vi "RQST Wait on Multiple Requests.vi"(6 "Processed Outgoing":refnum<queue>, 7 "Name":string, 8 "error in (no error)":errorcluster, 9 "value":T4[](array[typedef]), 10 "Source Address":u8=27, 11 "RQST ref":T3) -> (0 "error out":errorcluster, 1 "Global Requests":bool[](array[boolean]), 2 "Timeouts":bool[](array[boolean]), 3 "Elements":T1[](array[typedef]) {"payload" format="%x"; "timestamp" format="%<%.7X\n%x>T"; "type" items=["CAN Data"=0, "CAN Remote"=1, "CAN Bus Error"=2, "J1939 Data"=192, "Delay"=224, "Log Trigger"=225, "Start Trigger"=226]; "identifier" format="%x"})   [LabVIEW 2013, in "J1939.lvlib"]
uses:
  J1939.lvlib
  API Types/WS_Request Message.ctl
  RQST Lookup Table Reference.ctl
  <vilib>/xnet/xnet.llb/XNET Frame CAN.ctl
  <vilib>/xnet/xnet.llb/XNET Frame Type CAN.ctl
  API Types/CAN Outgoing Message Cluster.ctl
  RQST Lookup Table Cluster.ctl
  Common Messages/J1939 Message Request.vi
  Frame Conversion/Common Conversions.vi
  Frame Conversion/Convert J1939 ID to CAN Arb ID.vi
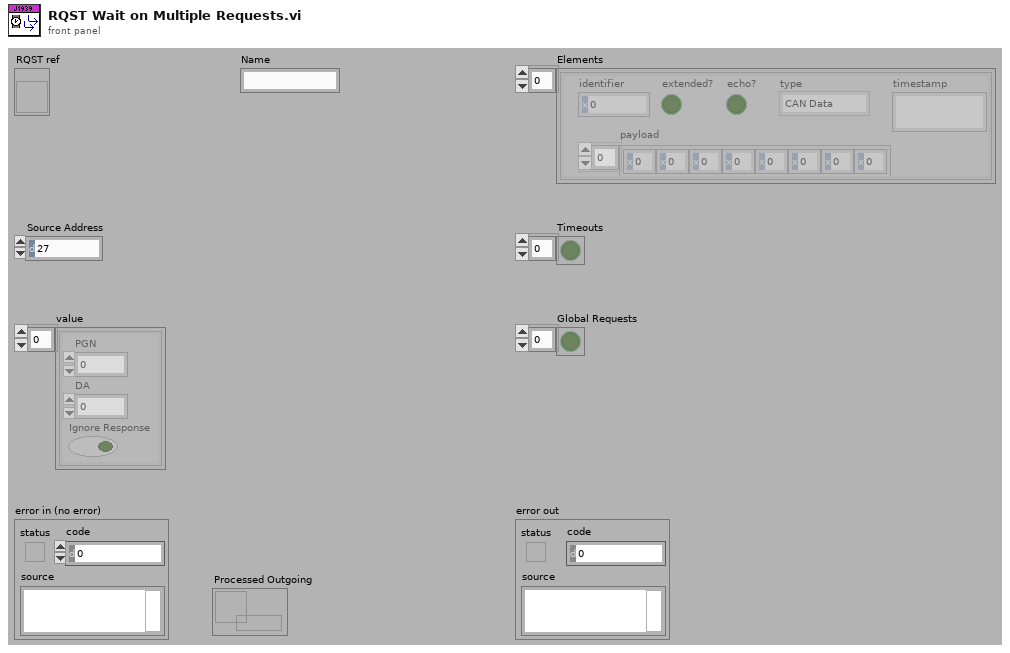
[diagram p1: front panel]
types:
  T1 = typedef "XNET Frame CAN.ctl" = cluster{"timestamp":timestamp, "payload":u8[], "identifier":u32, "type":T2, "extended?":bool, "echo?":bool}
  T2 = typedef "XNET Frame Type CAN.ctl" = u8
  T3 = typedef "J1939.lvlib/RQST Lookup Table Reference.ctl" = refnum<vi>
  T4 = typedef "J1939.lvlib/WS_Request Message.ctl" = cluster{"PGN":u32, "DA":u8, "Ignore Response":bool}
  T5 = typedef "J1939.lvlib/CAN Outgoing Message Cluster.ctl" = cluster{"Identifier":u32, "Data":u8[]}
  T6 = typedef "J1939.lvlib/RQST Lookup Table Cluster.ctl" = cluster{"Response Q":refnum<queue>, "Request PGN":u32}
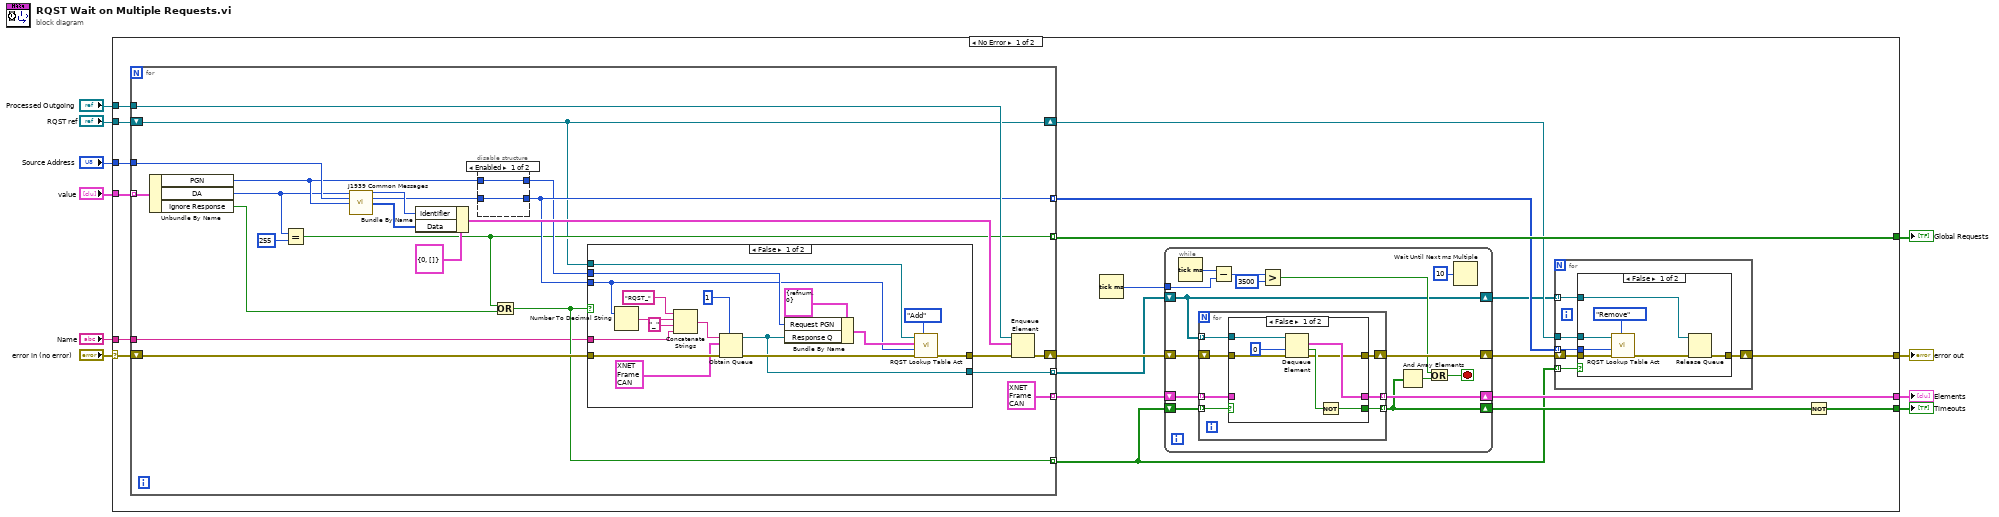
[diagram p0: block diagram]
diagram:
  n1 = case shown="No Error" "error in (no error)" {
    selector: "error in (no error)" -> [w30 w121]
    tunnel: "Source Address" -> [w25 _]
    tunnel: "RQST ref" -> [w17 _]
    tunnel: [w20 w121] -> w6
    tunnel: [w29 _] -> w8
    tunnel: [w15 _] -> w7
    tunnel: "Processed Outgoing" -> [w26 _]
    tunnel: [w24 _] -> w3
    tunnel: "value" -> [w23 _]
    tunnel: "Name" -> [w11 _]
    frame No Error {
      n2 = for {
        tunnel: [w98] -> w13 mode=indexing
        tunnel: w26 -> [w95]
        tunnel: [w89] -> w19 mode=indexing
        tunnel: w25 -> [w87]
        tunnel: [w85] -> w16 mode=indexing
        tunnel: [w84] -> w24 mode=indexing
        shift-right: [w96] -> w27
        shift-left: w30 -> [w99]
        tunnel: w23 -> [w83] mode=indexing
        shift-right: [w79] -> w18
        shift-left: w17 -> [w79]
        tunnel: [T1 {"timestamp"=timestamp(0 s since 1904-01-01), "payload"=[], "identifier"=0, "type"=0, "extended?"=FALSE, "echo?"=FALSE} ("CAN frame")] -> w12 mode=indexing
        tunnel: w11 -> [w77]
        n3 = Unbundle By Name(w83) -> ("PGN"=w82:u32, "DA"=w81:u8, "Ignore Response"=w80:bool)
        n4 = Equal?(x=w81, y=u8 255) -> (x = y?=w84:bool)
        n5 = call-poly "J1939 Common Messages.vi"("Destination Address"=w81, "Source Address"=w87, "PGN"=w82) -> ("Arb ID"=w92:u32, "Expected Return Arb ID"=w90:u32, "Data"=w93:u8[])  [unwired: 10 in]
        n6 = Bundle By Name(cluster=T5 {"Identifier"=0, "Data"=[]} ("element"), "Identifier"=w92, "Data"=w93) -> (w91:T5)
        n7 = disable-structure shown="Enabled" {
          disable-tunnel: [w119 w120] -> w89
          disable-tunnel: w90 -> [w119 _]
          disable-tunnel: w82 -> [w118 w120]
          disable-tunnel: [w118 w120] -> w88
          frame Enabled {
          }
          frame Disabled {
          }
        }
        n8 = Or(x=w84, y=w80) -> (x .or. y?=w85:bool)
        n9 = case shown="False" w85 {
          tunnel: w99 -> [w115 w117]
          tunnel: w79 -> [w109 _]
          tunnel: [w108 _] -> w98
          tunnel: [w107 w117] -> w97
          tunnel: w89 -> [w100 _]
          tunnel: w88 -> [w106 _]
          tunnel: w77 -> [w103 _]
          frame False {
            n10 = Number To Decimal String(number=w100) -> (decimal integer string=w101:string)  [unwired: 1 in]
            n11 = Concatenate Strings("RQST_" ("string"), w101, "_" ("string"), w103) -> (w102:string)
            n12 = Obtain Queue(max queue size (-1, unlimited)=1, name (unnamed)=w102, element data type=T1 {"timestamp"=timestamp(0 s since 1904-01-01), "payload"=[], "identifier"=0, "type"=0, "extended?"=FALSE, "echo?"=FALSE} ("CAN frame"), error in (no error)=w115) -> (queue out=w108:refnum<queue>, error out=w114:errorcluster)  [unwired: 1 in, 1 out]
            n13 = Bundle By Name(cluster=T6 {"Response Q"=refnum, "Request PGN"=0} ("Data"), "Request PGN"=w106, "Response Q"=w108) -> (w111:T6)
            n14 = call "RQST Lookup Table Act.vi"("Action"=enum16{"Initialize", "Add", "Get", "Remove"}."Add", "error in (no error)"=w114, "ID"=w100, "Data"=w111, "ref in"=w109) -> ("error out"=w107:errorcluster)  [unwired: 4 in, 2 out]
          }
          frame True {
          }
        }
        n15 = Enqueue Element(queue=w95, element=w91, error in (no error)=w97) -> (error out=w96:errorcluster)  [unwired: 1 in, 2 out]
      }
      n16 = Tick Count (ms)() -> (millisecond timer value=w22:u32)
      n17 = while {
        shift-right: [w58] -> w29
        shift-left: w12 -> [w55]
        shift-right: [w54] -> w28
        shift-left: w16 -> [w56]
        tunnel: w22 -> [w50]
        shift-right: [w59] -> w21
        shift-left: w27 -> [w57]
        shift-right: [w46] -> w14
        shift-left: w13 -> [w46]
        stop <- w52 stop-if-true
        n18 = Tick Count (ms)() -> (millisecond timer value=w51:u32)
        n19 = for {
          tunnel: w46 -> [w66] mode=indexing
          tunnel: [w64] -> w58 mode=indexing
          tunnel: [w63] -> w54 mode=indexing
          tunnel: w56 -> [w61] mode=indexing
          tunnel: w55 -> [w60] mode=indexing
          shift-right: [w65] -> w59
          shift-left: w57 -> [w62]
          n20 = case shown="False" w61 {
            selector: w61 -> [_ w75]
            tunnel: w66 -> [w72 _]
            tunnel: [w68 w76] -> w65
            tunnel: [w71 w74] -> w64
            tunnel: [w67 w75] -> w63
            tunnel: w62 -> [w69 w76]
            tunnel: w60 -> [_ w74]
            frame False {
              n21 = Dequeue Element(queue=w72, timeout in ms (-1)=0, error in (no error)=w69) -> (element=w71:T1, timed out?=w70:bool, error out=w68:errorcluster)  [unwired: 1 out]
              n22 = Not(x=w70) -> (.not. x?=w67:bool)
            }
            frame True {
            }
          }
        }
        n23 = Subtract(x=w51, y=w50) -> (x-y=w49:u32)
        n24 = Greater?(x=w49, y=u32 3500) -> (0:w47:bool)
        n25 = And Array Elements(Boolean array=w54) -> (logical AND=w53:bool)
        n26 = Or(x=w47, y=w53) -> (x .or. y?=w52:bool)
        n27 = Wait Until Next ms Multiple(millisecond multiple=u32 10) -> ()  [unwired: 1 out]
      }
      n28 = for {
        shift-right: [w35] -> w20
        shift-left: w21 -> [w36]
        tunnel: w14 -> [w34] mode=indexing
        tunnel: w19 -> [w33] mode=indexing
        tunnel: w18 -> [w32]
        tunnel: w16 -> [w31] mode=indexing
        n29 = case shown="False" w31 {
          tunnel: w32 -> [w43 _]
          tunnel: [w40 w44] -> w35
          tunnel: w36 -> [w37 w44]
          tunnel: w33 -> [w39 _]
          tunnel: w34 -> [w38 _]
          frame False {
            n30 = call "RQST Lookup Table Act.vi"("Action"=enum16{"Initialize", "Add", "Get", "Remove"}."Remove", "error in (no error)"=w37, "ID"=w39, "ref in"=w43) -> ("error out"=w41:errorcluster)  [unwired: 5 in, 2 out]
            n31 = Release Queue(queue=w38, error in (no error)=w41) -> (error out=w40:errorcluster)  [unwired: 1 in, 2 out]
          }
          frame True {
          }
        }
      }
      n32 = Not(x=w28) -> (.not. x?=w15:bool[])
    }
    frame Error {
    }
  }
  "Elements" <- w8
  "Timeouts" <- w7
  "error out" <- w6
  "Global Requests" <- w3
